vi "Write Spectrum.vi"(7 "Window Width":u32=10, 8 "error in (no error)":errorcluster, 9 "Depth":u32=50, 10 "Spectrum":dbl[](array[numeric]), 11 "Spectral Processing in":refnum<class "Spectral Processing.lvclass">) -> (0 "error out":errorcluster, 3 "Spectral Processing out":refnum<class "Spectral Processing.lvclass">)   [LabVIEW 2014, in "Spectral Processing.lvclass"]
uses:
  Spectral Processing.lvclass
  Spectral Processing.lvclass/Spectral Processing.ctl
  <vilib>/Analysis/baseanly.llb/Mean (DBL).vi
  <vilib>/Analysis/4window.llb/Hanning Window (DBL).vi
  <vilib>/Analysis/2dsp.llb/Real FFT.vi
  <vilib>/Analysis/4window.llb/AllCosWindow (DBL).vi
  <vilib>/Analysis/NI_AALPro.lvlib
  <vilib>/Analysis/NI_AALBase.lvlib
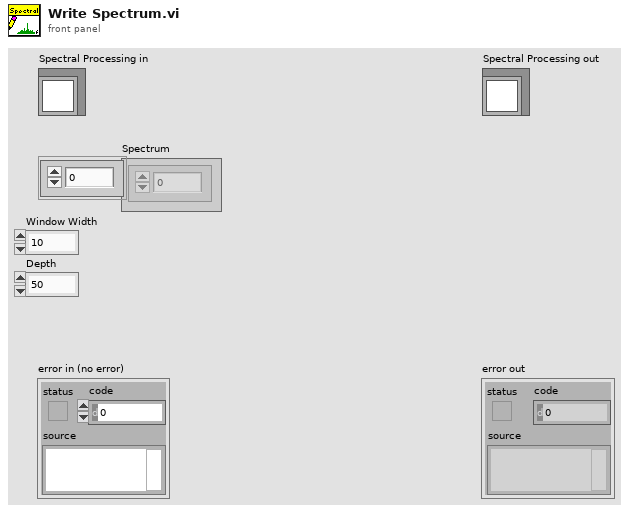
[diagram p1: front panel]
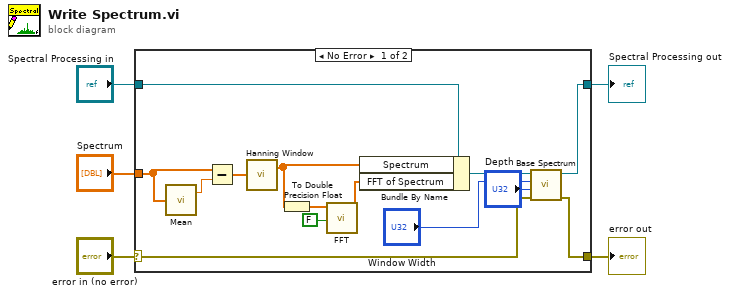
[diagram p0: block diagram]
diagram:
  n1 = case shown="No Error" "error in (no error)" {
    selector: "error in (no error)" -> [w16 w20]
    tunnel: [w15 w20] -> w4
    tunnel: [w17 w21] -> w2
    tunnel: "Spectral Processing in" -> [w19 w21]
    tunnel: "Spectrum" -> [w10 _]
    frame No Error {
      n2 = call-poly <vilib>:"Mean.vi"("X"=w10) -> ("mean"=w11:dbl)  [unwired: 1 out]
      n3 = Subtract(x=w10, y=w11) -> (x-y=w9:dbl[])
      n4 = call-poly <vilib>:"Hanning Window.vi"("X"=w9) -> ("Windowed X"=w8:dbl[])  [unwired: 1 out]
      n5 = To Double Precision Float(number=w8) -> (double precision float=w14:dbl[])
      n6 = call-poly <vilib>:"FFT.vi"("shift?"=FALSE, "X"=w14) -> ("FFT {X}"=w12:cdb[])  [unwired: 8 in, 1 out]
      n7 = Bundle By Name(cluster=w19, "Spectrum"=w8, "FFT of Spectrum"=w12) -> (w18:refnum<class "Spectral Processing.lvclass">)
      n8 = call "Base Spectrum.vi"("error in (no error)"=w16, "Depth"="Depth", "Window Width"="Window Width", "Spectral Processing in"=w18) -> ("error out"=w15:errorcluster, "Spectral Processing out"=w17:refnum<class "Spectral Processing.lvclass">)  [unwired: 6 in]
    }
    frame Error {
    }
  }
  "error out" <- w4
  "Spectral Processing out" <- w2
